vi "test PID angle.vi"() -> ()   [LabVIEW 2018]
uses:
  <vilib>/Analysis/coordinate.llb/Angle Range (Degree).ctl
  <vilib>/Analysis/coordinate.llb/Angle Units.ctl
  <vilib>/Analysis/coordinate.llb/Wrap Angle (scalar).vi
  <vilib>/Analysis/coordinate.llb/Angle Rotation (scalar).vi
  <vilib>/Analysis/coordinate.llb/Absolute Angle Difference (scalar).vi
  <vilib>/Analysis/coordinate.llb/Set Angle Unit.vi
  <vilib>/Analysis/NI_AAL_Angle.lvlib
panel:
  out "absolute angle difference":dbl
  out "T0":dbl
  out "set point":dbl
  in  "angle in 2":dbl
  in  "angle in":dbl
  in  "Rotation":dbl format="%#_13g"
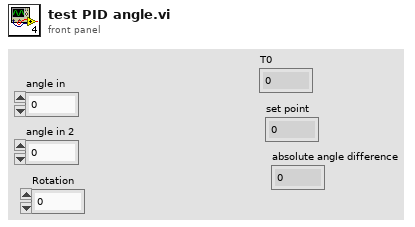
[diagram p1: front panel]
types:
  T1 = typedef "NI_AAL_Angle.lvlib/Angle Units.ctl" = i32
  T2 = typedef "NI_AAL_Angle.lvlib/Angle Range (Degree).ctl" = u16
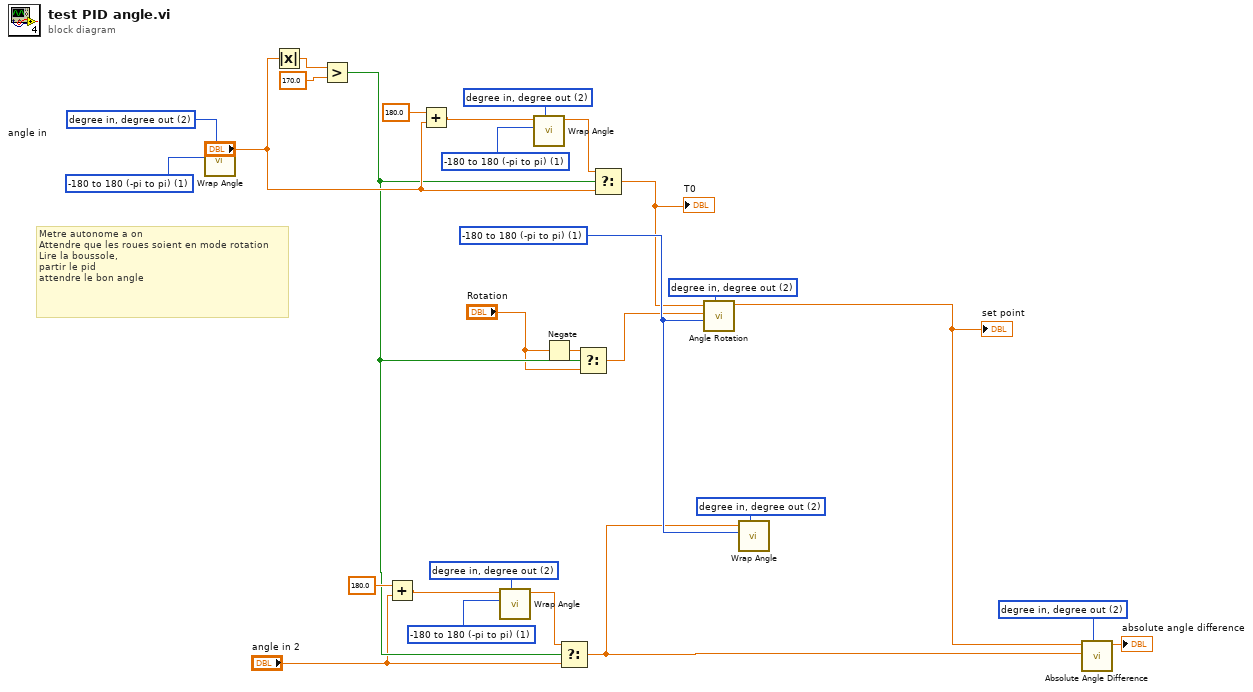
[diagram p0: block diagram]
diagram:
  w10 = T1 2 items=["radian in, radian out", "radian in, degree out", "degree in, degree out", "degree in, radian out"] ("angle units")
  w11 = T2 1 items=["none", "-180 to 180 (-pi to pi)", "0 to 360 (0 to 2pi)"] ("angle range")
  w20 = T1 2 items=["radian in, radian out", "radian in, degree out", "degree in, degree out", "degree in, radian out"] ("angle units")
  w19 = T2 1 items=["none", "-180 to 180 (-pi to pi)", "0 to 360 (0 to 2pi)"] ("angle range")
  w26 = T1 2 items=["radian in, radian out", "radian in, degree out", "degree in, degree out", "degree in, radian out"] ("angle units")
  w22 = T2 1 items=["none", "-180 to 180 (-pi to pi)", "0 to 360 (0 to 2pi)"] ("angle range")
  w29 = T2 1 items=["none", "-180 to 180 (-pi to pi)", "0 to 360 (0 to 2pi)"] ("angle range")
  w24 = T1 2 items=["radian in, radian out", "radian in, degree out", "degree in, degree out", "degree in, radian out"] ("angle units")
  w25 = T1 2 items=["radian in, radian out", "radian in, degree out", "degree in, degree out", "degree in, radian out"] ("angle units")
  w1 = T1 2 items=["radian in, radian out", "radian in, degree out", "degree in, degree out", "degree in, radian out"] ("angle units")
  # "Metre autonome a on\nAttendre que les roues soient en mode rotation\nLire la boussole,\npartir le pid\nattendre le bon angle"
  n1 = call-poly <vilib>:"Wrap Angle.vi"("angle units"=w26, "angle range"=w29, "angle in"="angle in") -> ("angle out"=w16:dbl)  [unwired: 7 in, 1 out]
  n2 = Absolute Value(x=w16) -> (abs(x)=w28:dbl)
  n3 = Greater?(x=w28, y=170.0) -> (0:w8:bool)
  n4 = Add(x=180.0, y="angle in 2") -> (x+y=w12:dbl)
  n5 = Add(x=180.0, y=w16) -> (x+y=w18:dbl)
  n6 = call-poly <vilib>:"Wrap Angle.vi"("angle units"=w10, "angle range"=w11, "angle in"=w12) -> ("angle out"=w13:dbl)  [unwired: 7 in, 1 out]
  n7 = call-poly <vilib>:"Wrap Angle.vi"("angle units"=w20, "angle range"=w19, "angle in"=w18) -> ("angle out"=w17:dbl)  [unwired: 7 in, 1 out]
  n8 = Negate(x="Rotation") -> (-x=w14:dbl)
  n9 = Select(t=w13, s=w8, f="angle in 2") -> (s? t:f=w4:dbl)
  n10 = Select(t=w14, s=w8, f="Rotation") -> (s? t:f=w5:dbl)
  n11 = Select(t=w17, s=w8, f=w16) -> (s? t:f=w15:dbl)
  "T0" <- w15
  n12 = call-poly <vilib>:"Angle Rotation.vi"("angle units"=w24, "rotated angle range"=w22, "counterclockwise rotation"=w5, "angle"=w15) -> ("rotated angle"=w3:dbl)  [unwired: 6 in, 1 out]
  "set point" <- w3
  n13 = call-poly <vilib>:"Wrap Angle.vi"("angle units"=w25, "angle range"=w22, "angle in"=w4) -> ()  [unwired: 7 in, 2 out]
  n14 = call-poly <vilib>:"Absolute Angle Difference.vi"("angle units"=w1, "angle 2"=w4, "angle 1"=w3) -> ("absolute angle difference"=→"absolute angle difference":dbl)  [unwired: 7 in, 1 out]
